vi "Populate Tree.vi"(6 "New root item?":refnum<vi>, 7 "Indent level":i32, 8 "error in":errorcluster, 9 "Data in":string[](array[string]), 10 "Tags map":refnum<vi>, 11 "TreeControl in":refnum<vi>) -> (0 "error out":errorcluster)   [LabVIEW 2025, in "CAN-LIN Raw Bus Capture UI.lvlib"]
doc: "This VI adds each data row to the tree. Gives back the SIGNALS table data."
uses:
  CAN-LIN Raw Bus Capture UI.lvlib
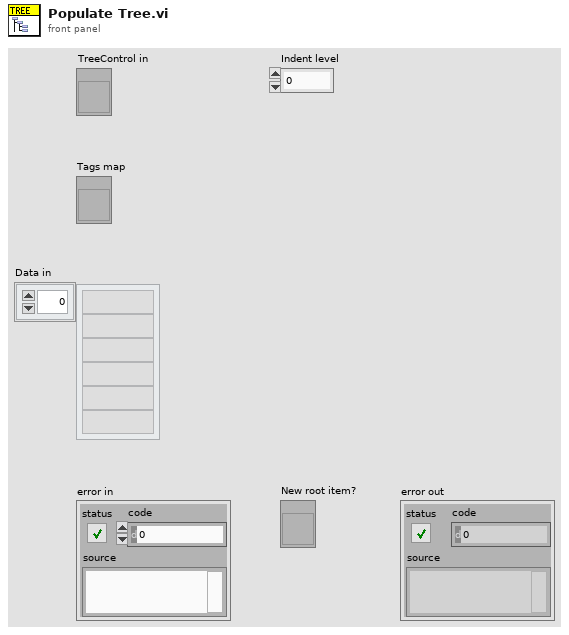
[diagram p1: front panel]
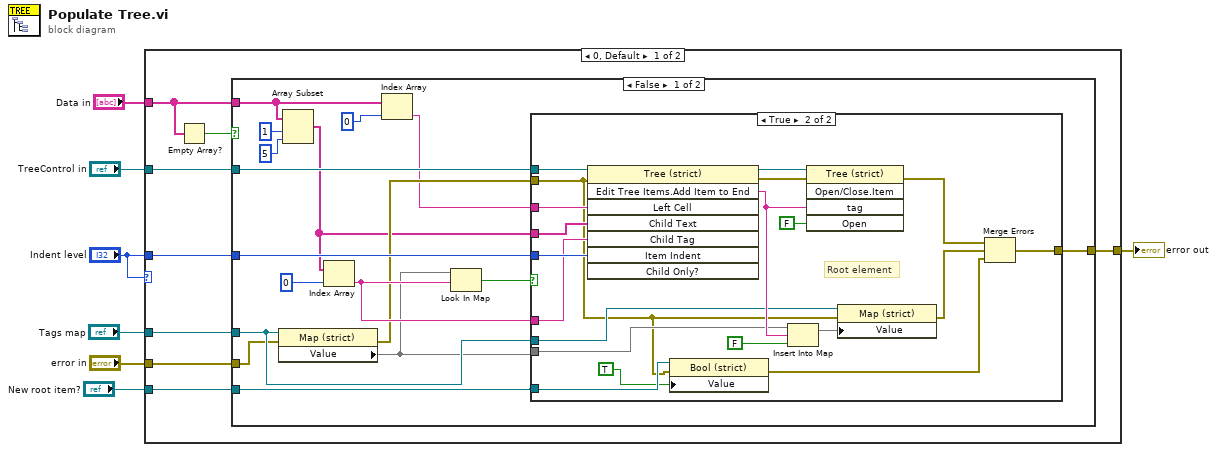
[diagram p0: block diagram]
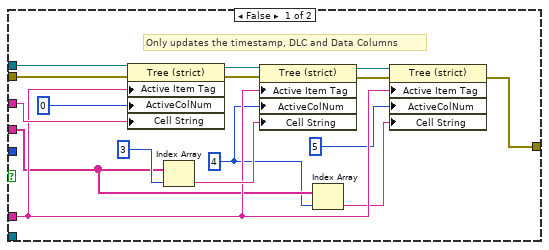
[diagram p2: hidden frame]
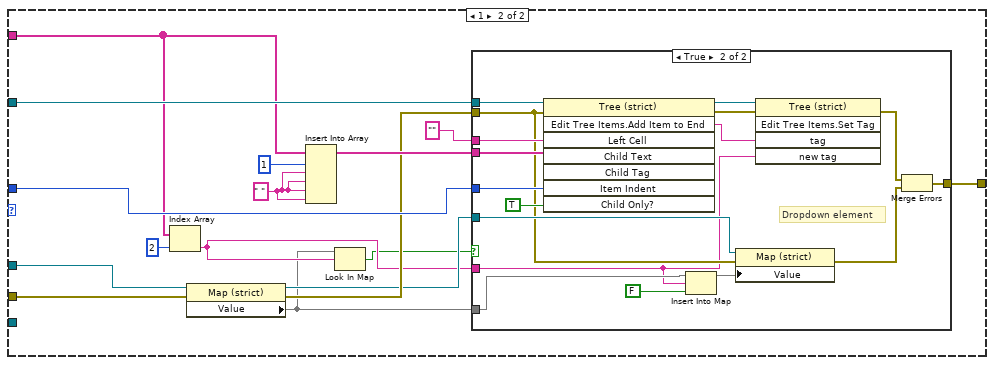
[diagram p4: hidden frame]
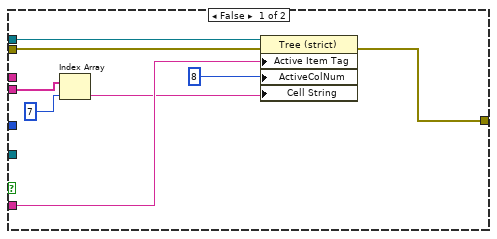
[diagram p5: hidden frame]
diagram:
  n1 = case shown="0, Default" "Indent level" {
    tunnel: "Indent level" -> [w15 w85]
    tunnel: [w14 w84] -> w7
    tunnel: "TreeControl in" -> [w12 w79]
    tunnel: "error in" -> [w11 w77]
    tunnel: "Tags map" -> [w13 w78]
    tunnel: "Data in" -> [w9 w71]
    tunnel: "New root item?" -> [w10 _]
    frame 0, Default {
      n2 = Empty Array?(array=w9) -> (empty?=w8:bool)
      n3 = case shown="False" w8 {
        tunnel: w15 -> [w32 _]
        tunnel: [w31 w69] -> w14
        tunnel: w13 -> [w29 _]
        tunnel: w12 -> [w27 _]
        tunnel: w11 -> [w26 w69]
        tunnel: w9 -> [w19 _]
        tunnel: w10 -> [w16 _]
        frame False {
          n4 = property class="Map (strict)"(reference=w29, error in=w26) -> (error out=w25:errorcluster, "Value"=w23:map{string, bool})  [unwired: 1 out]
          n5 = Array Subset(array=w19, index=1, length=5) -> (w18:string[])
          n6 = Index Array(array=w18, index=0) -> (element=w28:string)
          n7 = Index Array(array=w19, index=0) -> (element=w17:string)
          n8 = Look In Map(map=w23, key=w28) -> (key not found?=w24:bool)  [unwired: 1 in, 1 out]
          n9 = case shown="True" w24 {
            tunnel: w27 -> [w48 w65]
            tunnel: w25 -> [w47 w50]
            tunnel: w32 -> [_ w64]
            tunnel: [w35 w55] -> w31
            tunnel: w17 -> [w45 w63]
            tunnel: w18 -> [w37 w62]
            tunnel: w28 -> [w38 w61]
            tunnel: w29 -> [_ w54]
            tunnel: w23 -> [_ w53]
            tunnel: w16 -> [_ w52]
            frame False {
              w34 = 4 ("index")
              # "Only updates the timestamp, DLC and Data Columns"
              n10 = property class="Tree (strict)"(reference=w48, error in=w47, "Active Item Tag"=w38, "ActiveColNum"=0 ("Active Cell:Active Column Number"), "Cell String"=w45) -> (reference out=w44:refnum<vi>, error out=w43:errorcluster)
              n11 = Index Array(array=w37, index=3 ("Active Cell:Active Column Number")) -> (element=w41:string)
              n12 = property class="Tree (strict)"(reference=w44, error in=w43, "Active Item Tag"=w38, "ActiveColNum"=w34, "Cell String"=w41) -> (reference out=w40:refnum<vi>, error out=w39:errorcluster)
              n13 = Index Array(array=w37, index=w34) -> (element=w36:string)
              n14 = property class="Tree (strict)"(reference=w40, error in=w39, "Active Item Tag"=w38, "ActiveColNum"=5 ("Active Cell:Active Column Number"), "Cell String"=w36) -> (error out=w35:errorcluster)  [unwired: 1 out]
            }
            frame True {
              # "Root element"
              n15 = invoke on="Invoke Node" class="Tree (strict)" method="Edit Tree Items.Add Item to End"(reference=w65, error in=w50, "Left Cell"=w63, "Child Text"=w62, "Child Tag"=w61, "Item Indent"=w64) -> (reference out=w66:refnum<vi>, error out=w68:errorcluster, "Edit Tree Items:Add Item to End"=w60:string)  [unwired: 2 in, 5 out]
              n16 = property class="Bool (strict)"(reference=w52, error in=w50, "Value"=TRUE) -> (error out=w49:errorcluster)  [unwired: 1 out]
              n17 = Insert Into Map(map in=w53, key=w60, value=FALSE) -> (map out=w58:map{string, bool})  [unwired: 2 out]
              n18 = invoke on="Invoke Node" class="Tree (strict)" method="Open/Close.Item"(reference=w66, error in=w68, "tag"=w60, "Open"=FALSE ("Open?")) -> (error out=w57:errorcluster)  [unwired: 1 in, 4 out]
              n19 = property class="Map (strict)"(reference=w54, error in=w50, "Value"=w58) -> (error out=w56:errorcluster)  [unwired: 1 out]
              n20 = Merge Errors(w57, w56, w49) -> (w55:errorcluster)
            }
          }
        }
        frame True {
        }
      }
    }
    frame 1 {
      w81 = " " ("new element/subarray")
      n21 = Index Array(array=w71, index=2) -> (element=w74:string)
      n22 = property class="Map (strict)"(reference=w78, error in=w77) -> (reference out=w75:refnum<vi>, error out=w76:errorcluster, "Value"=w73:map{string, bool})
      n23 = Insert Into Array(array=w71, index=1, new element #1=w81, new element #2=w81, new element #3=w81, new element #4=w81) -> (w82:string[])
      n24 = Look In Map(map=w73, key=w74) -> (key not found?=w72:bool)  [unwired: 1 in, 1 out]
      n25 = case shown="True" w72 {
        tunnel: w85 -> [_ w110]
        tunnel: [w93 w95] -> w84
        tunnel: "" ("Timestamp") -> [_ w109]
        tunnel: w82 -> [w88 w105]
        tunnel: w79 -> [w91 w104]
        tunnel: w74 -> [w92 w94]
        tunnel: w76 -> [w90 w98]
        tunnel: w73 -> [_ w100]
        tunnel: w75 -> [_ w99]
        frame False {
          n26 = Index Array(array=w88, index=7) -> (element=w86:string)
          n27 = property class="Tree (strict)"(reference=w91, error in=w90, "Active Item Tag"=w92, "ActiveColNum"=8 ("Active Cell:Active Column Number"), "Cell String"=w86) -> (error out=w93:errorcluster)  [unwired: 1 out]
        }
        frame True {
          # "Dropdown element"
          n28 = invoke on="Invoke Node" class="Tree (strict)" method="Edit Tree Items.Add Item to End"(reference=w104, error in=w98, "Left Cell"=w109, "Child Text"=w105, "Item Indent"=w110, "Child Only?"=TRUE) -> (reference out=w106:refnum<vi>, error out=w107:errorcluster, "Edit Tree Items:Add Item to End"=w108:string)  [unwired: 2 in, 5 out]
          n29 = Insert Into Map(map in=w100, key=w94, value=FALSE) -> (map out=w101:map{string, bool})  [unwired: 2 out]
          n30 = property class="Map (strict)"(reference=w99, error in=w98, "Value"=w101) -> (error out=w97:errorcluster)  [unwired: 1 out]
          n31 = invoke on="Invoke Node" class="Tree (strict)" method="Edit Tree Items.Set Tag"(reference=w106, error in=w107, "tag"=w108, "new tag"=w94) -> (error out=w96:errorcluster)  [unwired: 1 in, 4 out]
          n32 = Merge Errors(w96, w97) -> (w95:errorcluster)
        }
      }
    }
  }
  "error out" <- w7
